vi "Init Control.vi"(5 "Group":refnum<class "Group.lvclass">, 7 "VolatusAPI":refnum<class "VolatusAPI.lvclass">, 8 "error in (no error)":errorcluster, 9 "Control MsgQ":refnum<class "MessageQ.lvclass">, 10 "Config Element":refnum<class "Config Element.lvclass">, 11 "PulsedValve in":refnum<class "PulsedValve.lvclass">) -> (0 "error out":errorcluster, 3 "PulsedValve out":refnum<class "PulsedValve.lvclass">)   [LabVIEW 2020, in "VolatusControl.lvlib" / "PulsedValve.lvclass"]
uses:
  PulsedValve.lvclass
  lv-cdm/CDM-Config/Config Element/Config Element.lvclass
  Volatus/VolatusAPI/VolatusAPI.lvclass
  Volatus/MessageQ/MessageQ.lvclass
  PulsedValve.lvclass/PulsedValve.ctl
  lv-cdm/CDM-Config/Config Filter/Config Lookup.lvclass
  lv-vecto/Vecto/GroupAbstract/GroupAbstract.lvclass
  lv-vecto/Vecto/Group/Group.lvclass
  C:/dev/lv20CE/relink/lv-vecto/Vecto/GroupAbstract/GroupAbstract.lvclass
  C:/dev/lv20CE/relink/lv-vecto/Vecto/Group/Group.lvclass
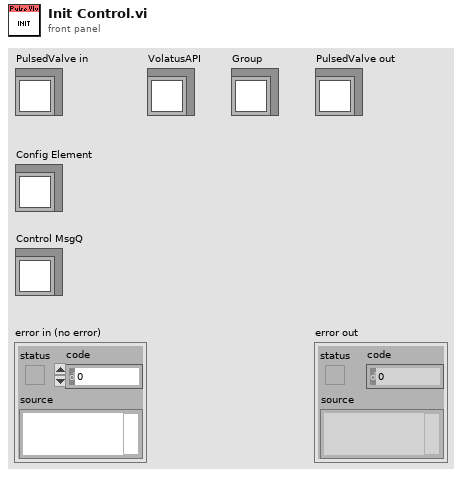
[diagram p1: front panel]
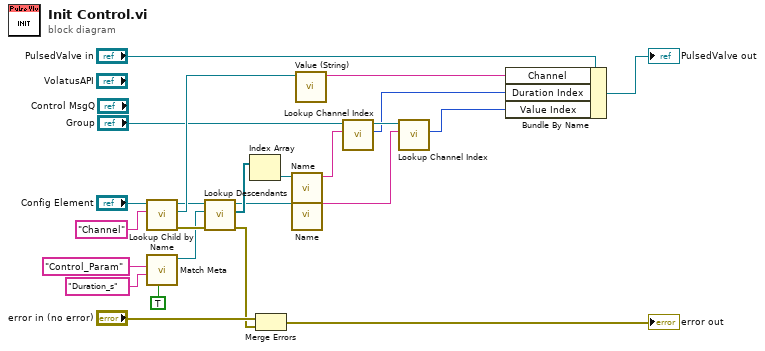
[diagram p0: block diagram]
diagram:
  n1 = call "Lookup Child by Name.vi"("Name"="Channel", "Config Element in"="Config Element") -> ("error out"=w15:errorcluster, "Child"=w19:refnum<class "Config Element.lvclass">, "Config Element out"=w16:refnum<class "Config Element.lvclass">)  [unwired: 6 in, 1 out]
  n2 = call "Match Meta.vi"("Exact Value (F)"=TRUE, "Value (Any)"="Duration_s" ("Name"), "Name"="Control_Param") -> ("Config Lookup out"=w14:refnum<class "Config Lookup.lvclass">)  [unwired: 7 in, 1 out]
  n3 = call "Lookup Descendants.vi"("error in (no error)"=w15, "Lookup"=w14, "Config Element in"=w16) -> ("error out"=w10:errorcluster, "Descendants"=w13:refnum<class "Config Element.lvclass">[], "Config Element out"=w8:refnum<class "Config Element.lvclass">)  [unwired: 6 in]
  n4 = Index Array(array=w13) -> (element=w7:refnum<class "Config Element.lvclass">)  [unwired: 1 in]
  n5 = Merge Errors("error in (no error)", w10) -> (→"error out":errorcluster)
  n6 = call "Name.vi"("Config Element in"=w7) -> ("Name"=w5:string)  [unwired: 9 in, 1 out]
  n7 = call "Name.vi"("Config Element in"=w8) -> ("Name"=w2:string)  [unwired: 9 in, 1 out]
  n8 = call "Value (String).vi"("Config Element in"=w19) -> ("String Value"=w12:string)  [unwired: 9 in, 1 out]
  n9 = call "Lookup Channel Index.vi"("Channel Name"=w5, "GroupAbstract in"="Group") -> ("Index"=w3:i32, "GroupAbstract out"=w4:refnum<class "Group.lvclass">)  [unwired: 7 in, 1 out]
  n10 = call "Lookup Channel Index.vi"("Channel Name"=w2, "GroupAbstract in"=w4) -> ("Index"=w1:i32)  [unwired: 7 in, 2 out]
  n11 = Bundle By Name(cluster="PulsedValve in", "Channel"=w12, "Duration Index"=w3, "Value Index"=w1) -> (→"PulsedValve out":refnum<class "PulsedValve.lvclass">)
